vi "ExecuteGrSimTestAttacker.vi"(0 "RandomAllyPoints":dbl[][](array[numeric]), 1 "IA State Input":T3, 2 "Modulo Velocidade":dbl format="%#_13g", 5 "id":i32, 7 "RandomEnemyPoints":dbl[][](array[numeric]), 9 "reset":bool, 11 "Test Mode On":bool, 12 "Replace Robots":bool, 14 "Number of Points":i32) -> (4 "grSim replacement":cluster{"robots":T1[], "ball":T2}={"robots"=[{"x"=0.0, "y"=-450.0, "dir"=0.0, "yellowteam"=FALSE, "id"=0}, {"x"=0.0, "y"=-270.0, "dir"=0.0, "yellowteam"=FALSE, "id"=1}, {"x"=0.0, "y"=-90.0, "dir"=0.0, "yellowteam"=FALSE, "id"=2}, {"x"=0.0, "y"=90.0, "dir"=0.0, "yellowteam"=FALSE, "id"=3}, {"x"=0.0, "y"=270.0, "dir"=0.0, "yellowteam"=FALSE, "id"=4}, {"x"=0.0, "y"=450.0, "dir"=0.0, "yellowteam"=FALSE, "id"=5}], "ball"={"x"=0.0, "y"=0.0, "vx"=0.0, "vy"=0.0}}, 6 "Replace active":bool, 8 "kick num":i32)   [LabVIEW 2017]
uses:
  Core/AI Input.ctl
  Core/AI Robot.ctl
  Intel/Functions Enum.ctl
  Intel/AttackerStates.ctl
  Path Planning/RRT/PathDests.ctl
  Path Planning/RRT/PathDest.ctl
  Core/AI Ball.ctl
  Core/Field Size.ctl
  Core/AI Judge.ctl
  Intel/Command Enum.ctl
  Util/Events/Events.ctl
  grSim RobotReplacement.ctl
  grSim_BallReplacement.ctl
panel:
  in  "Time":enum16{"Azul", "Amarelo"}(ring) caption="Enum"
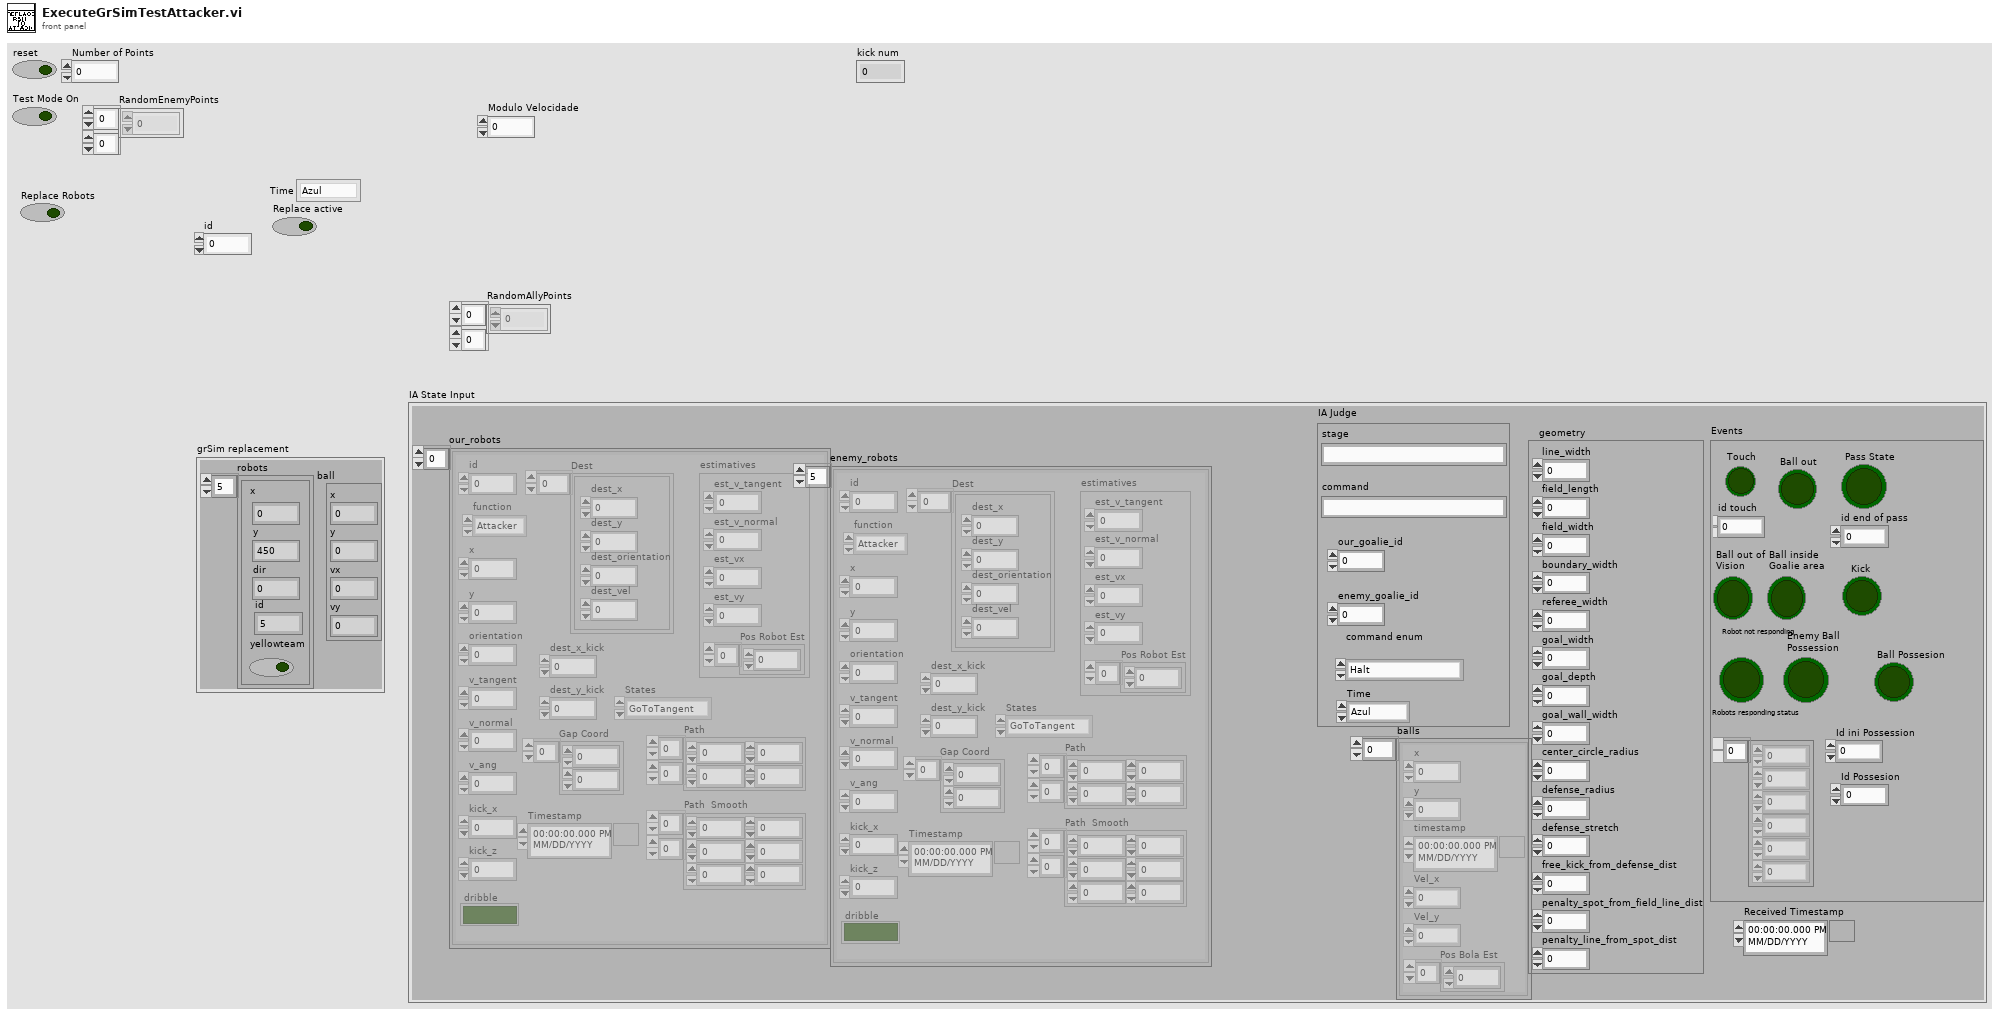
[diagram p1: front panel]
types:
  T1 = typedef "grSim RobotReplacement.ctl" = cluster{"x":dbl, "y":dbl, "dir":dbl, "yellowteam":bool, "id":u32}
  T2 = typedef "grSim_BallReplacement.ctl" = cluster{"x":dbl, "y":dbl, "vx":dbl, "vy":dbl}
  T3 = typedef "AI Input.ctl" = cluster{"our_robots":T4[], "enemy_robots":T4[], "balls":T9[], "geometry":T10, "IA Judge":T11, "Received Timestamp":timestamp, "Events":T13}
  T4 = typedef "AI Robot.ctl" = cluster{"id":u32, "function":T5, "x":dbl, "y":dbl, "orientation":dbl, "v_tangent":dbl, "v_normal":dbl, "v_ang":dbl, "kick_x":dbl, "kick_z":dbl, "dribble":bool, "Timestamp":timestamp, "estimatives":cluster{"est_v_tangent":dbl, "est_v_normal":dbl, "est_vx":dbl, "est_vy":dbl, "Pos Robot Est":dbl[]}, "dest_x_kick":dbl, "dest_y_kick":dbl, "Gap Coord":dbl[], "States":T6, "Path ":dbl[][], "Path  Smooth":dbl[][], "Dest":T7}
  T5 = typedef "Functions Enum.ctl" = enum16{"Attacker", "Goalie", "Defender", "Striker", "Goto 0", "Dummy", "Kicker", "ZigZag"}
  T6 = typedef "AttackerStates.ctl" = enum16{"Pass", "GoToTangent", "BallGetting", "GoToKick", ""}
  T7 = typedef "PathDests.ctl" = T8[]
  T8 = typedef "PathDest.ctl" = cluster{"dest_x":dbl, "dest_y":dbl, "dest_orientation":dbl, "dest_vel":dbl}
  T9 = typedef "AI Ball.ctl" = cluster{"x":dbl, "y":dbl, "timestamp":timestamp, "Vel_x":dbl, "Vel_y":dbl, "Pos Bola Est":dbl[]}
  T10 = typedef "Field Size.ctl" = cluster{"line_width":u32, "field_length":u32, "field_width":u32, "boundary_width":u32, "referee_width":u32, "goal_width":u32, "goal_depth":u32, "goal_wall_width":u32, "center_circle_radius":u32, "defense_radius":u32, "defense_stretch":u32, "free_kick_from_defense_dist":u32, "penalty_spot_from_field_line_dist":u32, "penalty_line_from_spot_dist":u32}
  T11 = typedef "AI Judge.ctl" = cluster{"stage":string, "command":string, "our_goalie_id":dbl, "enemy_goalie_id":dbl, "command enum":T12, "Time":enum16{"Azul", "Amarelo"}}
  T12 = typedef "Command Enum.ctl" = enum16{"Halt", "Stop", "Force Start", "PKA Normal Start", "Prepare Kickoff Ally", "PKE Normal Start", "Prepare Kickoff Enemy", "Prepare Penalty Ally", "PPA Normal Start", "Prepare Penalty Enemy", "PPE Normal Start", "Direct Free Enemy", "Direct Free Ally", "Indirect Free Enemy", "Indirect Free Ally", "Timeout Enemy", "Timeout Ally", "Goal Enemy", "Goal Ally", "Ball Placement Enemy", "Ball Placement Ally", "Normal Half Time", "Extra Time Break", "Extra Half Time", "None", "Post Game"}
  T13 = typedef "Events.ctl" = cluster{"Touch":bool, "Ball out":bool, "id touch":dbl, "Ball out of \nVision":bool, "Ball inside \nGoalie area":bool, "Robot not responding":bool, "Robots responding status":dbl[], "Enemy Ball \nPossession":bool, "Pass State":bool, "id end of pass":dbl, "Kick":bool, "Id ini Possession":dbl, "Ball Possesion":bool, "Id Possesion":dbl}
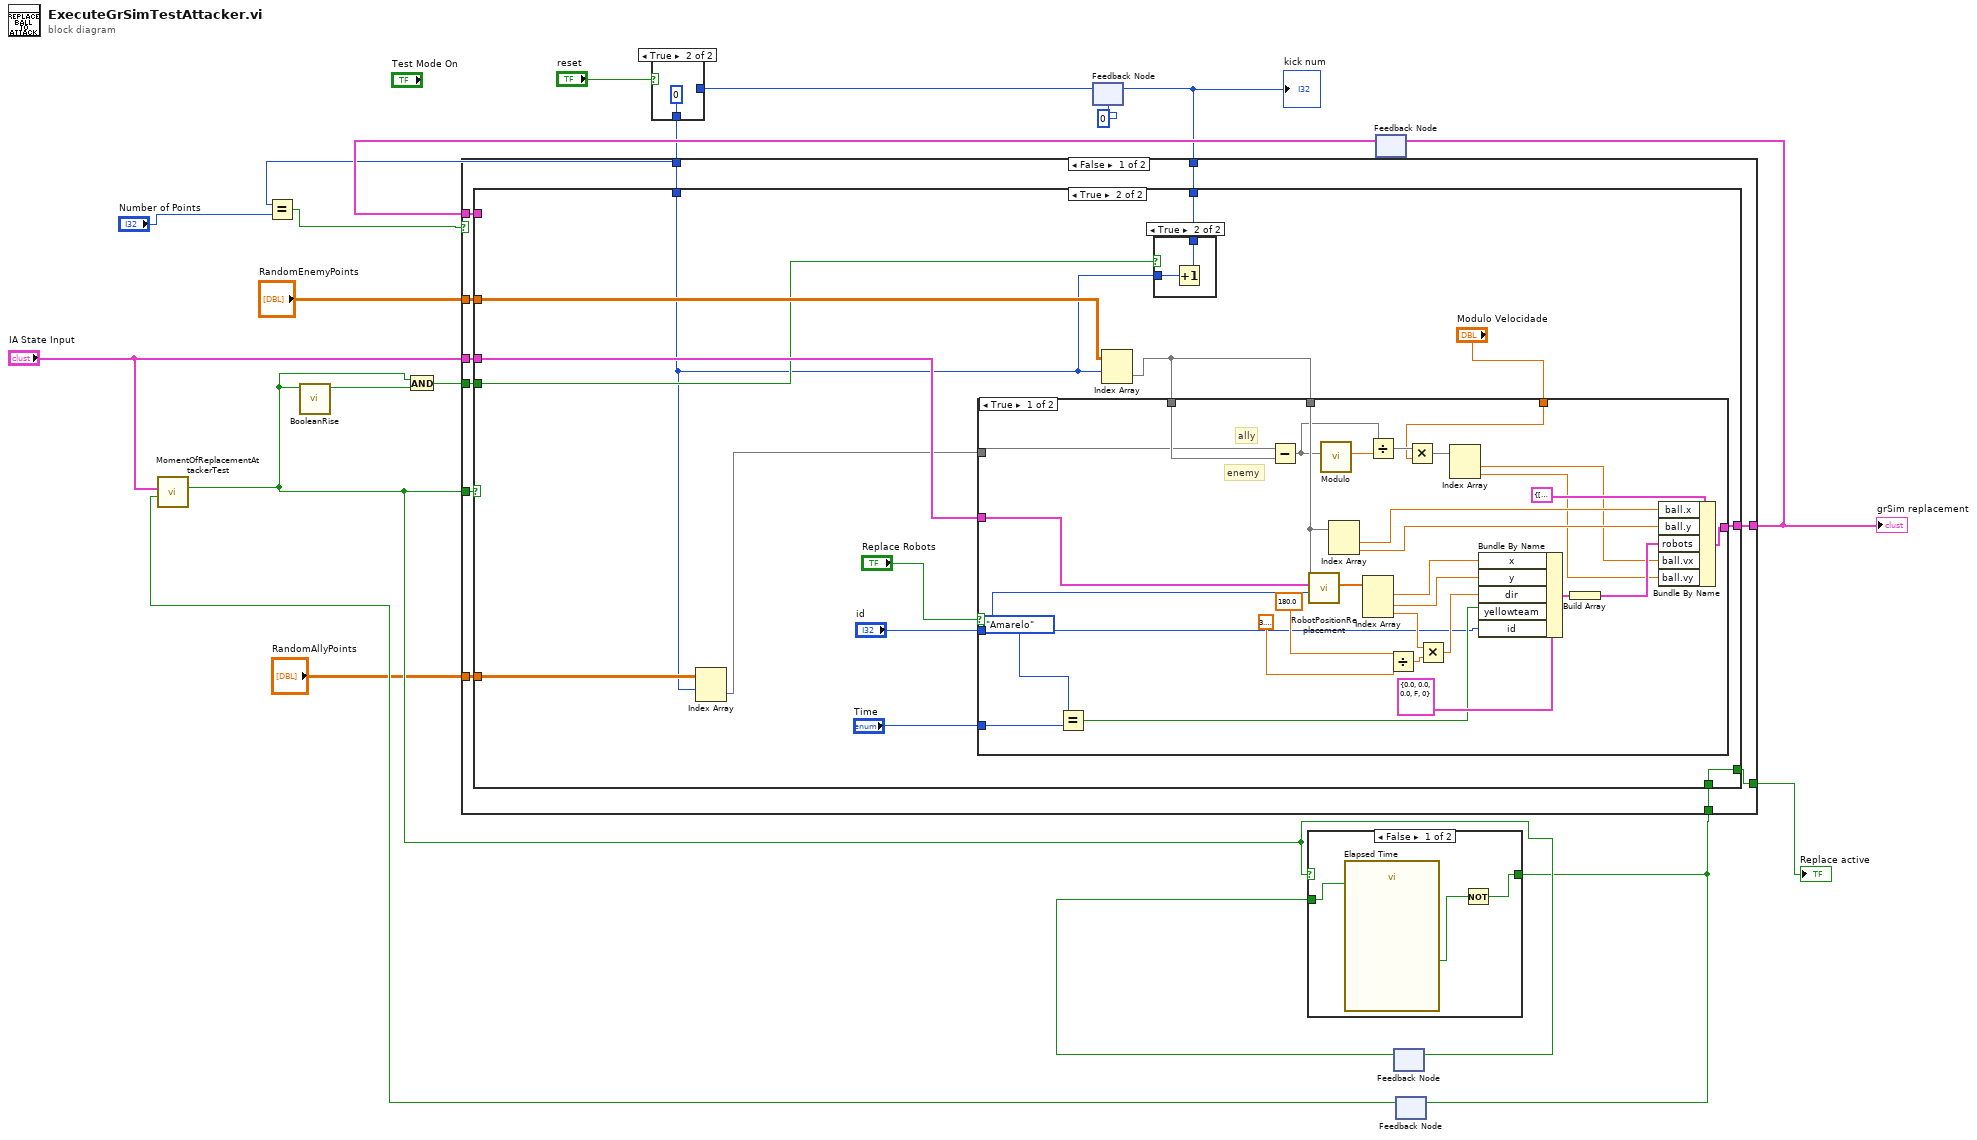
[diagram p0: block diagram]
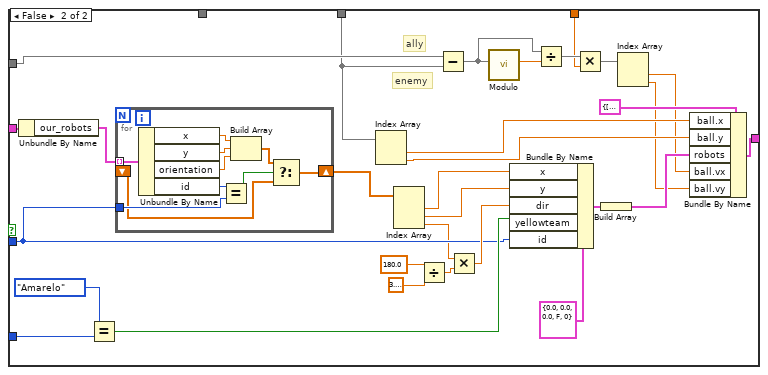
[diagram p4: hidden frame]
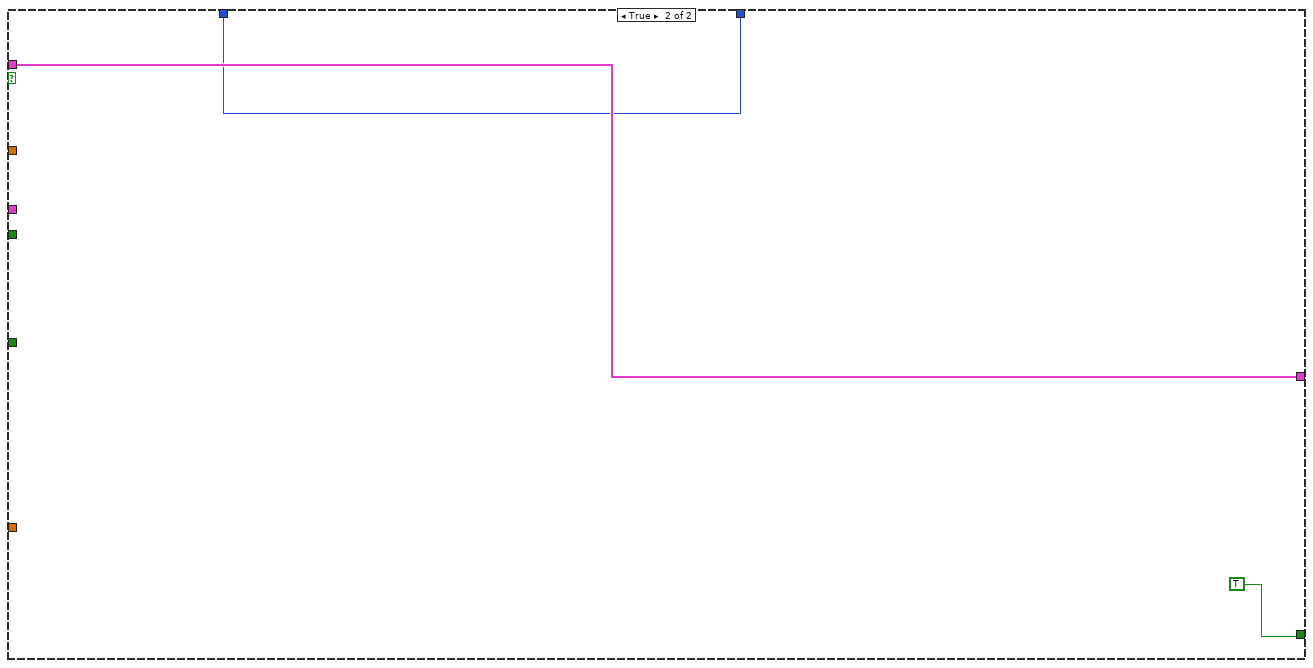
[diagram p5: hidden frame]
diagram:
  n1 = feedback #1(0) -> (w8:i32)
  n2 = case shown="True" "reset" {
    tunnel: w8 -> [w20 _]
    tunnel: [w20 0] -> w5
    frame False {
    }
    frame True {
    }
  }
  n3 = Equal?(x=w5, y="Number of Points") -> (x = y?=w4:bool)
  n4 = feedback #2() -> (w19:cluster{"robots":T1[], "ball":T2})  [unwired: 1 in]
  n5 = feedback #3() -> (w18:bool)  [unwired: 1 in]
  n6 = feedback #4() -> (w15:bool)  [unwired: 1 in]
  n7 = call "MomentOfReplacementAttackerTest.vi"("Replace active"=w15, "IA State Input"="IA State Input") -> ("Time to replace?"=w9:bool)  [unwired: 9 in]
  n8 = call "BooleanRise.vi"("Test Mode On"=w9) -> ("Boolean"=w10:bool)  [unwired: 10 in]
  n9 = And(x=w9, y=w10) -> (x .and. y?=w11:bool)
  n10 = case shown="False" w9 {
    selector: w9 -> [_ w25]
    tunnel: [w24 w25] -> w3
    tunnel: w18 -> [w22 _]
    frame False {
      n11 = call "Elapsed Time"("Reset"=w22) -> ("Time has Elapsed"=w23:bool)  [unwired: 11 in, 7 out]
      n12 = Not(x=w23) -> (.not. x?=w24:bool)
    }
    frame True {
    }
  }
  n13 = case shown="False" w4 {
    tunnel: w19 -> [w36 w128]
    tunnel: [w35 w128] -> w17
    tunnel: "IA State Input" -> [w34 _]
    tunnel: "RandomEnemyPoints" -> [w33 _]
    tunnel: [w32 w127] -> w12
    tunnel: w11 -> [w31 _]
    tunnel: w9 -> [w30 _]
    tunnel: w5 -> [w29 w127]
    tunnel: w3 -> [w27 _]
    tunnel: [w28 TRUE] -> w2
    tunnel: "RandomAllyPoints" -> [w26 _]
    frame False {
      n14 = case shown="True" w30 {
        tunnel: [w39 w53] -> w35
        tunnel: w34 -> [_ w51]
        tunnel: w36 -> [w39 _]
        tunnel: w33 -> [_ w50]
        tunnel: w29 -> [w38 w43]
        tunnel: [w38 w47] -> w32
        tunnel: w31 -> [_ w46]
        tunnel: [w37 w45] -> w28
        tunnel: w27 -> [w37 w45]
        tunnel: w26 -> [_ w44]
        frame False {
        }
        frame True {
          n15 = Index Array(array=w44, index (row)=w43) -> (element=w42:dbl[])  [unwired: 1 in]
          n16 = Index Array(array=w50, index (row)=w43) -> (element=w41:dbl[])  [unwired: 1 in]
          n17 = case shown="True" "Replace Robots" {
            tunnel: [w86 w116] -> w53
            tunnel: w41 -> [w69 w94]
            tunnel: "Time" -> [w82 w112]
            tunnel: w51 -> [w77 w105]
            tunnel: "id" -> [w70 w103]
            tunnel: w42 -> [w60 w95]
            tunnel: w41 -> [w61 _]
            tunnel: "Modulo Velocidade" -> [w57 w87]
            frame True {
              # "enemy"
              # "ally"
              n18 = Equal?(x=enum16{"Azul", "Amarelo"}."Amarelo", y=w82) -> (x = y?=w80:bool)
              n19 = Subtract(x=w60, y=w61) -> (x-y=w63:dbl[])
              n20 = call "RobotPositionReplacement.vi"("id"=w70, "IA State Input"=w77, "Position Ball"=w69) -> ("Position Robot"=w79:dbl[])  [unwired: 6 in]
              n21 = call "Modulo.vi"("2D vector"=w63) -> ("Modulo"=w62:dbl)  [unwired: 10 in]
              n22 = Index Array(array=w69) -> (element #1=w68:dbl, element #2=w67:dbl)  [unwired: 2 in]
              n23 = Index Array(array=w79) -> (element #1=w78:dbl, element #2=w76:dbl, element #3=w71:dbl)  [unwired: 3 in]
              n24 = Divide(x=w63, y=w62) -> (x/y=w64:dbl[])
              n25 = Divide(x=180.0, y=3.141592653589793) -> (x/y=w74:dbl)
              n26 = Multiply(x=w64, y=w57) -> (x*y=w65:dbl[])
              n27 = Multiply(x=w71, y=w74) -> (x*y=w75:dbl)
              n28 = Index Array(array=w65) -> (element #1=w59:dbl, element #2=w58:dbl)  [unwired: 2 in]
              n29 = Bundle By Name(cluster=T1 {"x"=0.0, "y"=0.0, "dir"=0.0, "yellowteam"=FALSE, "id"=0} ("element"), "x"=w78, "y"=w76, "dir"=w75, "yellowteam"=w80, "id"=w70) -> (w84:T1)
              n30 = Build Array(w84) -> (w83:T1[])
              n31 = Bundle By Name(cluster=cluster{"robots":T1[], "ball":T2} {"robots"=[{"x"=0.0, "y"=-450.0, "dir"=0.0, "yellowteam"=FALSE, "id"=0}, {"x"=0.0, "y"=-270.0, "dir"=0.0, "yellowteam"=FALSE, "id"=1}, {"x"=0.0, "y"=-90.0, "dir"=0.0, "yellowteam"=FALSE, "id"=2}, {"x"=0.0, "y"=90.0, "dir"=0.0, "yellowteam"=FALSE, "id"=3}, {"x"=0.0, "y"=270.0, "dir"=0.0, "yellowteam"=FALSE, "id"=4}, {"x"=0.0, "y"=450.0, "dir"=0.0, "yellowteam"=FALSE, "id"=5}], "ball"={"x"=0.0, "y"=0.0, "vx"=0.0, "vy"=0.0}} ("grSim replacement"), "ball.x"=w68, "ball.y"=w67, "robots"=w83, "ball.vx"=w59, "ball.vy"=w58) -> (w86:cluster{"robots":T1[], "ball":T2})
            }
            frame False {
              # "enemy"
              # "ally"
              n32 = Unbundle By Name(w105) -> ("our_robots"=w104:T4[])
              n33 = Equal?(x=enum16{"Azul", "Amarelo"}."Amarelo", y=w112) -> (x = y?=w110:bool)
              n34 = for {
                tunnel: w104 -> [w126] mode=indexing
                tunnel: w103 -> [w124]
                shift-right: [w118] -> w102
                shift-left: _ -> [w117]
                n35 = Unbundle By Name(w126) -> ("x"=w123:dbl, "y"=w122:dbl, "orientation"=w121:dbl, "id"=w125:u32)
                n36 = Equal?(x=w125, y=w124) -> (x = y?=w120:bool)
                n37 = Build Array(w123, w122, w121) -> (w119:dbl[])
                n38 = Select(t=w119, s=w120, f=w117) -> (s? t:f=w118:dbl[])
              }
              n39 = Index Array(array=w94) -> (element #1=w98:dbl, element #2=w97:dbl)  [unwired: 2 in]
              n40 = Index Array(array=w102) -> (element #1=w101:dbl, element #2=w99:dbl, element #3=w100:dbl)  [unwired: 3 in]
              n41 = Divide(x=180.0, y=3.141592653589793) -> (x/y=w108:dbl)
              n42 = Subtract(x=w95, y=w94) -> (x-y=w92:dbl[])
              n43 = Multiply(x=w100, y=w108) -> (x*y=w109:dbl)
              n44 = call "Modulo.vi"("2D vector"=w92) -> ("Modulo"=w93:dbl)  [unwired: 10 in]
              n45 = Bundle By Name(cluster=T1 {"x"=0.0, "y"=0.0, "dir"=0.0, "yellowteam"=FALSE, "id"=0} ("element"), "x"=w101, "y"=w99, "dir"=w109, "yellowteam"=w110, "id"=w103) -> (w114:T1)
              n46 = Divide(x=w92, y=w93) -> (x/y=w91:dbl[])
              n47 = Multiply(x=w91, y=w87) -> (x*y=w90:dbl[])
              n48 = Build Array(w114) -> (w113:T1[])
              n49 = Index Array(array=w90) -> (element #1=w89:dbl, element #2=w88:dbl)  [unwired: 2 in]
              n50 = Bundle By Name(cluster=cluster{"robots":T1[], "ball":T2} {"robots"=[{"x"=0.0, "y"=-450.0, "dir"=0.0, "yellowteam"=FALSE, "id"=0}, {"x"=0.0, "y"=-270.0, "dir"=0.0, "yellowteam"=FALSE, "id"=1}, {"x"=0.0, "y"=-90.0, "dir"=0.0, "yellowteam"=FALSE, "id"=2}, {"x"=0.0, "y"=90.0, "dir"=0.0, "yellowteam"=FALSE, "id"=3}, {"x"=0.0, "y"=270.0, "dir"=0.0, "yellowteam"=FALSE, "id"=4}, {"x"=0.0, "y"=450.0, "dir"=0.0, "yellowteam"=FALSE, "id"=5}], "ball"={"x"=0.0, "y"=0.0, "vx"=0.0, "vy"=0.0}} ("grSim replacement"), "ball.x"=w98, "ball.y"=w97, "robots"=w113, "ball.vx"=w89, "ball.vy"=w88) -> (w116:cluster{"robots":T1[], "ball":T2})
            }
          }
          n51 = case shown="True" w46 {
            tunnel: w43 -> [w54 w56]
            tunnel: [w54 w55] -> w47
            frame False {
            }
            frame True {
              n52 = Increment(x=w56) -> (x+1=w55:i32)
            }
          }
        }
      }
    }
    frame True {
    }
  }
  "grSim replacement" <- w17
  "Replace active" <- w2
  "kick num" <- w12
  n53 = feedback-in #1(w12) -> ()
  n54 = feedback-in #2(w17) -> ()
  n55 = feedback-in #3(w9) -> ()
  n56 = feedback-in #4(w3) -> ()
